vi "SIM past outputs to BDs.vi"(11 "Array of previous outputs":dbl[][](array[numeric])=[[1.0], [2.0], [3.0]]) -> (3 "Corresponding backward differences":dbl[][](array[numeric])=[[1.0], [-1.0], [0.0]])   [LabVIEW 2018]
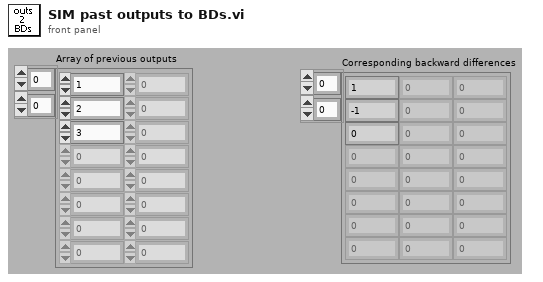
[diagram p1: front panel]
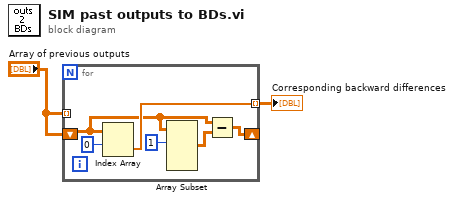
[diagram p0: block diagram]
diagram:
  n1 = for {
    shift-right: [w3] -> _
    shift-left: "Array of previous outputs" -> [w5]
    tunnel: [w7] -> w2 mode=indexing
    tunnel: "Array of previous outputs" -> [_] mode=indexing
    n2 = Index Array(array=w5, index (row)=0 ("index")) -> (element=w7:dbl[])  [unwired: 1 in]
    n3 = Array Subset(array=w5, index (row)=1 ("index")) -> (w6:dbl[][])  [unwired: 3 in]
    n4 = Subtract(x=w5, y=w6) -> (x-y=w3:dbl[][])
  }
  "Corresponding backward differences" <- w2
